vi "update.vi"(8 "error in (no error)":errorcluster, 9 "Actuate Settings":T1, 10 "ILC in":refnum<class "ILC.lvclass">, 11 "IActuator in":refnum<class "IActuator.lvclass">) -> (0 "error out":errorcluster, 2 "ILC out":refnum<class "ILC.lvclass">, 3 "IActuator out":refnum<class "IActuator.lvclass">)   [LabVIEW 2015, in "IActuator.lvclass"]
uses:
  IActuator.lvclass
  Typedefs/Actuate Settings.ctl
  Typedefs/ControlMode.ctl
  <userlib>/Common/ILC/ILC/ILC.lvclass
  Typedefs/FAMTTypedefs.lvlib
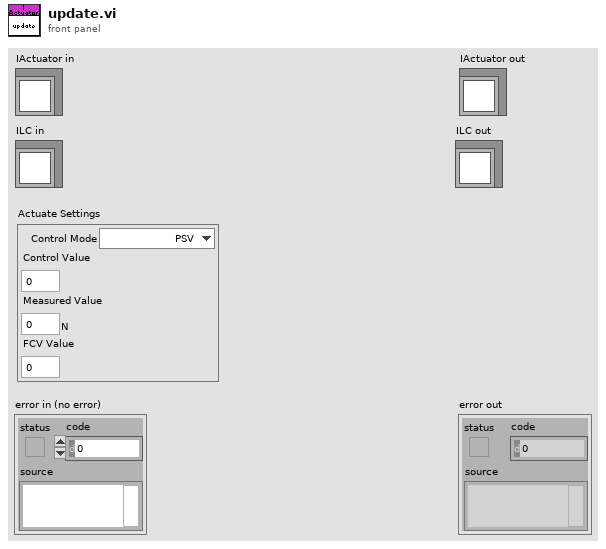
[diagram p1: front panel]
types:
  T1 = typedef "FAMTTypedefs.lvlib/Actuate Settings.ctl" = cluster{"Control Mode":T2, "Control Value":dbl, "Measured Value":dbl[unit], "FCV Value":dbl}
  T2 = typedef "FAMTTypedefs.lvlib/ControlMode.ctl" = enum16{"PSV", "FCV", "Both"}
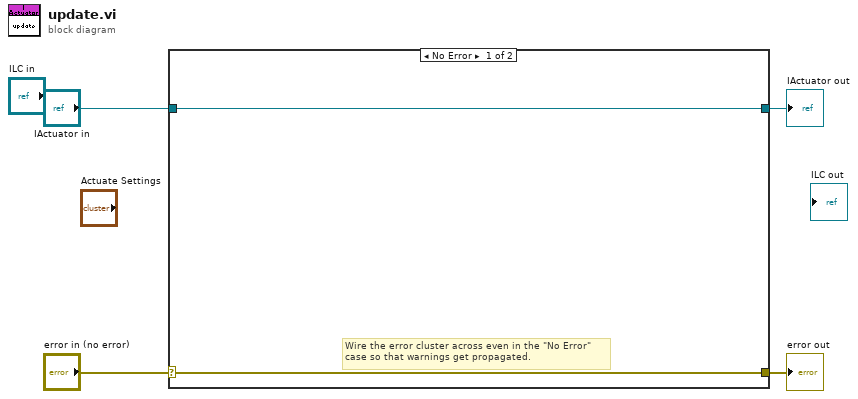
[diagram p0: block diagram]
diagram:
  n1 = case shown="No Error" "error in (no error)" {
    selector: "error in (no error)" -> [w5 w8]
    tunnel: [w5 w8] -> w3
    tunnel: [w6 w7] -> w1
    tunnel: "IActuator in" -> [w6 w7]
    frame No Error {
      # "Wire the error cluster across even in the \"No Error\"\ncase so that warnings get propagated."
    }
    frame Error {
    }
  }
  "error out" <- w3
  "IActuator out" <- w1
